vi "Caption Set Temperature.vi"(0 "Reference Cluster":T1) -> ()   [LabVIEW 2017, in "GUI.lvlib"]
uses:
  GUI.lvlib
  Konfiguracja/Konfiguracja.lvlib
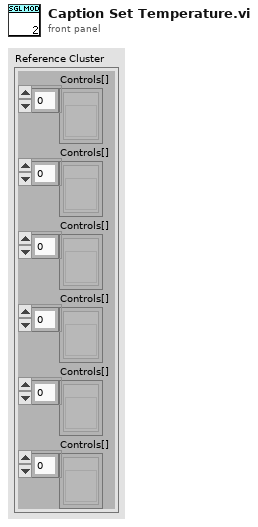
[diagram p1: front panel]
types:
  T1 = cluster{"Controls[]":refnum<vi>[], "Controls[]":refnum<vi>[], "Controls[]":refnum<vi>[], "Controls[]":refnum<vi>[], "Controls[]":refnum<vi>[], "Controls[]":refnum<vi>[]}
  T2 = cluster{"Termometr 1":string, "Termometr 2":string, "Termometr 3":string, "Termometr 4":string, "Termometr 5":string, "Termometr 6":string, "Termometr 7":string, "Termometr 8":string, "Termometr 9":string, "Termometr 10":string}
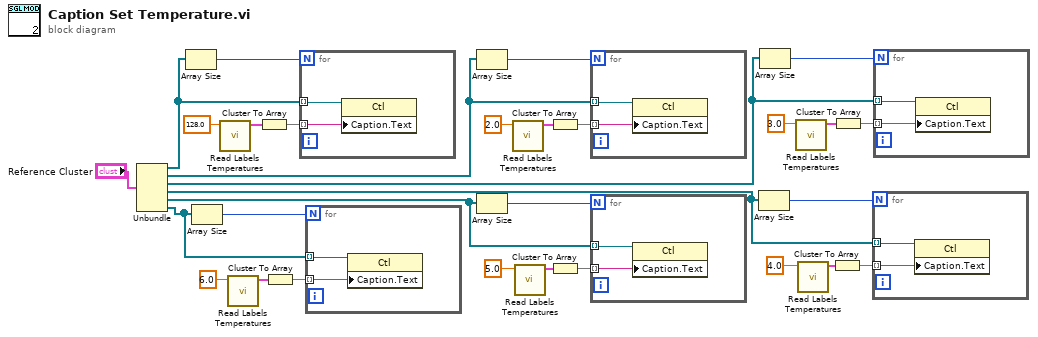
[diagram p0: block diagram]
diagram:
  n1 = Unbundle("Reference Cluster") -> ("Controls[]"=w30:refnum<vi>[], "Controls[]"=w25:refnum<vi>[], "Controls[]"=w22:refnum<vi>[], "Controls[]"=w19:refnum<vi>[], "Controls[]"=w16:refnum<vi>[], "Controls[]"=w13:refnum<vi>[])
  n2 = Array Size(array=w30) -> (size(s)=w29:i32)
  n3 = Array Size(array=w13) -> (size(s)=w15:i32)
  n4 = call "Read Labels Temperatures.vi"("Slave ID"=128.0) -> ("Etykiety T1-10"=w12:T2)  [unwired: 10 in]
  n5 = call "Read Labels Temperatures.vi"("Slave ID"=6.0) -> ("Etykiety T1-10"=w2:T2)  [unwired: 10 in]
  n6 = Cluster To Array(cluster=w12) -> (array=w28:string[])
  n7 = Cluster To Array(cluster=w2) -> (array=w14:string[])
  n8 = for {
    N: w29 -> [_]
    tunnel: w30 -> [w33] mode=indexing
    tunnel: w28 -> [w32] mode=indexing
    n9 = property class="Ctl"(reference=w33, "Caption.Text"=w32) -> ()  [unwired: 1 in, 2 out]
  }
  n10 = for {
    N: w15 -> [_]
    tunnel: w13 -> [w35] mode=indexing
    tunnel: w14 -> [w34] mode=indexing
    n11 = property class="Ctl"(reference=w35, "Caption.Text"=w34) -> ()  [unwired: 1 in, 2 out]
  }
  n12 = Array Size(array=w25) -> (size(s)=w27:i32)
  n13 = Array Size(array=w16) -> (size(s)=w18:i32)
  n14 = call "Read Labels Temperatures.vi"("Slave ID"=2.0) -> ("Etykiety T1-10"=w10:T2)  [unwired: 10 in]
  n15 = call "Read Labels Temperatures.vi"("Slave ID"=5.0) -> ("Etykiety T1-10"=w4:T2)  [unwired: 10 in]
  n16 = Cluster To Array(cluster=w10) -> (array=w26:string[])
  n17 = Cluster To Array(cluster=w4) -> (array=w17:string[])
  n18 = for {
    N: w27 -> [_]
    tunnel: w25 -> [w37] mode=indexing
    tunnel: w26 -> [w36] mode=indexing
    n19 = property class="Ctl"(reference=w37, "Caption.Text"=w36) -> ()  [unwired: 1 in, 2 out]
  }
  n20 = for {
    N: w18 -> [_]
    tunnel: w16 -> [w39] mode=indexing
    tunnel: w17 -> [w38] mode=indexing
    n21 = property class="Ctl"(reference=w39, "Caption.Text"=w38) -> ()  [unwired: 1 in, 2 out]
  }
  n22 = Array Size(array=w19) -> (size(s)=w21:i32)
  n23 = Array Size(array=w22) -> (size(s)=w24:i32)
  n24 = call "Read Labels Temperatures.vi"("Slave ID"=3.0) -> ("Etykiety T1-10"=w8:T2)  [unwired: 10 in]
  n25 = call "Read Labels Temperatures.vi"("Slave ID"=4.0) -> ("Etykiety T1-10"=w6:T2)  [unwired: 10 in]
  n26 = Cluster To Array(cluster=w6) -> (array=w20:string[])
  n27 = Cluster To Array(cluster=w8) -> (array=w23:string[])
  n28 = for {
    N: w21 -> [_]
    tunnel: w19 -> [w41] mode=indexing
    tunnel: w20 -> [w40] mode=indexing
    n29 = property class="Ctl"(reference=w41, "Caption.Text"=w40) -> ()  [unwired: 1 in, 2 out]
  }
  n30 = for {
    N: w24 -> [_]
    tunnel: w22 -> [w43] mode=indexing
    tunnel: w23 -> [w42] mode=indexing
    n31 = property class="Ctl"(reference=w43, "Caption.Text"=w42) -> ()  [unwired: 1 in, 2 out]
  }
